vi "Periodic Tasks.vi"(8 "error in":errorcluster) -> ()   [LabVIEW 2015]
doc: "This VI runs in parallel to other tasks. It can contain as many user-defined periodic loops as you need. These can carry out PID or other sorts of timed response."
uses:
  <vilib>/Rock Robotics/SystemInterfaces/Utilities/FPGA_UtilitiesLED Source.ctl
  <vilib>/Rock Robotics/SystemInterfaces/Utilities/FPGA_UtilitiesLED State.ctl
  Robot Global Data.vi
  <vilib>/Rock Robotics/WPI/Solenoid/WPI_SolenoidValue.ctl
  <vilib>/Rock Robotics/WPI/Solenoid/WPI_SolenoidSetEnum.vi
panel:
  out "Enabled":bool
  out "Compressor Running":bool
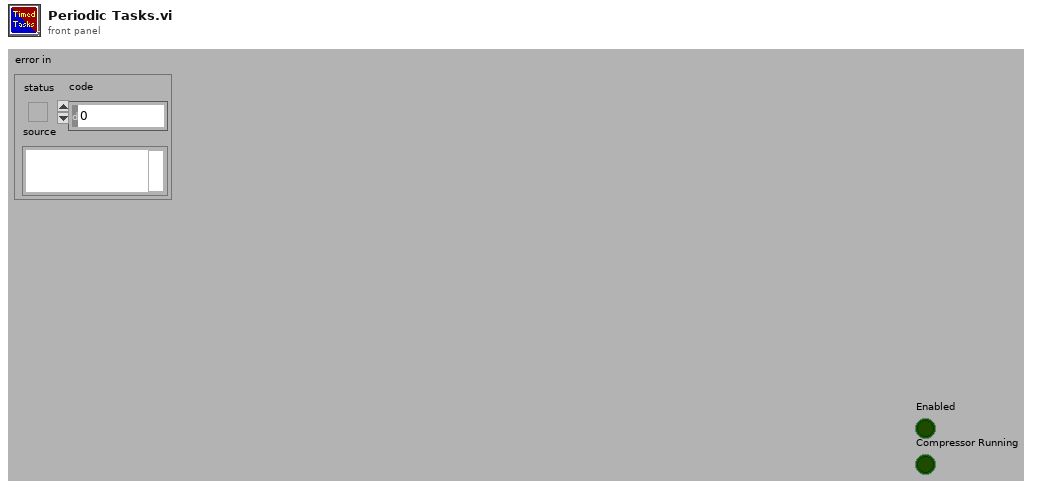
[diagram p1: front panel]
types:
  T1 = typedef "FPGA_UtilitiesLED State.ctl" = enum16{"Off", "On", "Toggle"}
  T2 = typedef "FPGA_UtilitiesLED Source.ctl" = enum16{"User LED", "FPGA LED"}
  T3 = typedef "WPI_MotorControlDeviceRef.ctl" = cluster{"DeviceStatus":errorcluster, "Type":enum16{"PWM", "CAN"}, "PWM":cluster{"Digital Module":T4, "PWM Channel":T5, "DeadBand":T6}, "CAN":cluster{"Device Number":u8, "Control Mode":T7, "Semaphore":T8, "Max Vout":dbl}, "Invert":bool, "TransformRef":T9, "InvTransformRef":T9}
  T4 = typedef "FPGA_TypedefDigitalModule.ctl" = enum16{"Digital Module 1", "Digital Module 2"}
  T5 = typedef "FPGA_DIOPWMChannel.ctl" = enum8{"PWM 1", "PWM 2", "PWM 3", "PWM 4", "PWM 5", "PWM 6", "PWM 7", "PWM 8", "PWM 9", "PWM 10", "Invalid"}
  T6 = typedef "WPI_PWMDeadband.ctl" = cluster{"Name":string, "maxPositivePwm":i32, "minPositivePwm":i32, "centerPwm":i32, "maxNegativePwm":i32, "minNegativePwm":i32, "angularRange":u16}
  T7 = typedef "WPI_CANJaguar_ControlMode.ctl" = enum8{"Percent VBus", "Current", "Speed", "Position", "Voltage"}
  T8 = typedef "Semaphore RefNum" = refnum<k1>
  T9 = typedef "WPI_PWMTransform_ConPane.ctl" = refnum<vi>
  T10 = typedef "WPI_SolenoidValue.ctl" = enum16{"Off", "On", "Forward", "Reverse"}
  T11 = typedef "WPI_SolenoidDevRef.ctl" = cluster{"DevStatus":errorcluster, "Solenoid Module":T12, "Forward Solenoid Channel":T13, "Reverse Solenoid Channel":T13}
  T12 = typedef "FPGA_TypedefSolenoidModule.ctl" = enum16{"Solenoid Module 1", "Solenoid Module 2"}
  T13 = typedef "WPI_SolenoidChannel.ctl" = enum8{"Solenoid 1", "Solenoid 2", "Solenoid 3", "Solenoid 4", "Solenoid 5", "Solenoid 6", "Solenoid 7", "Solenoid 8", "Invalid"}
  T14 = typedef "WPI_DriverStationRobotMode2.ctl" = enum16{"Autonomous Disabled", "Autonomous Enabled", "Teleop Disabled", "Teleop Enabled", "Disconnected", "Finish", "Test Disabled", "Test Enabled"}
  T15 = typedef "WPI_CompressorDevRef.ctl" = cluster{"DevStatus":errorcluster, "DigitalInputDevRef":T16, "RelayDevRef":T18}
  T16 = typedef "WPI_DigitalInputDevRef.ctl" = cluster{"DevStatus":errorcluster, "DIO Channel":T17, "Digital Module":T4}
  T17 = typedef "FPGA_DIOChannel.ctl" = enum8{"DIO 1", "DIO 2", "DIO 3", "DIO 4", "DIO 5", "DIO 6", "DIO 7", "DIO 8", "DIO 9", "DIO 10", "DIO 11", "DIO 12", "DIO 13", "DIO 14", "Invalid"}
  T18 = typedef "WPI_RelayDevRef.ctl" = cluster{"DevStatus":errorcluster, "Relay Channel":T19, "Digital Module":T4, "Relay Direction":T20}
  T19 = typedef "FPGA_DIORelayChannel.ctl" = enum8{"Relay 1", "Relay 2", "Relay 3", "Relay 4", "Relay 5", "Relay 6", "Relay 7", "Relay 8", "Invalid"}
  T20 = typedef "WPI_RelayDirection.ctl" = enum16{"Both directions", "Forward only", "Reverse only"}
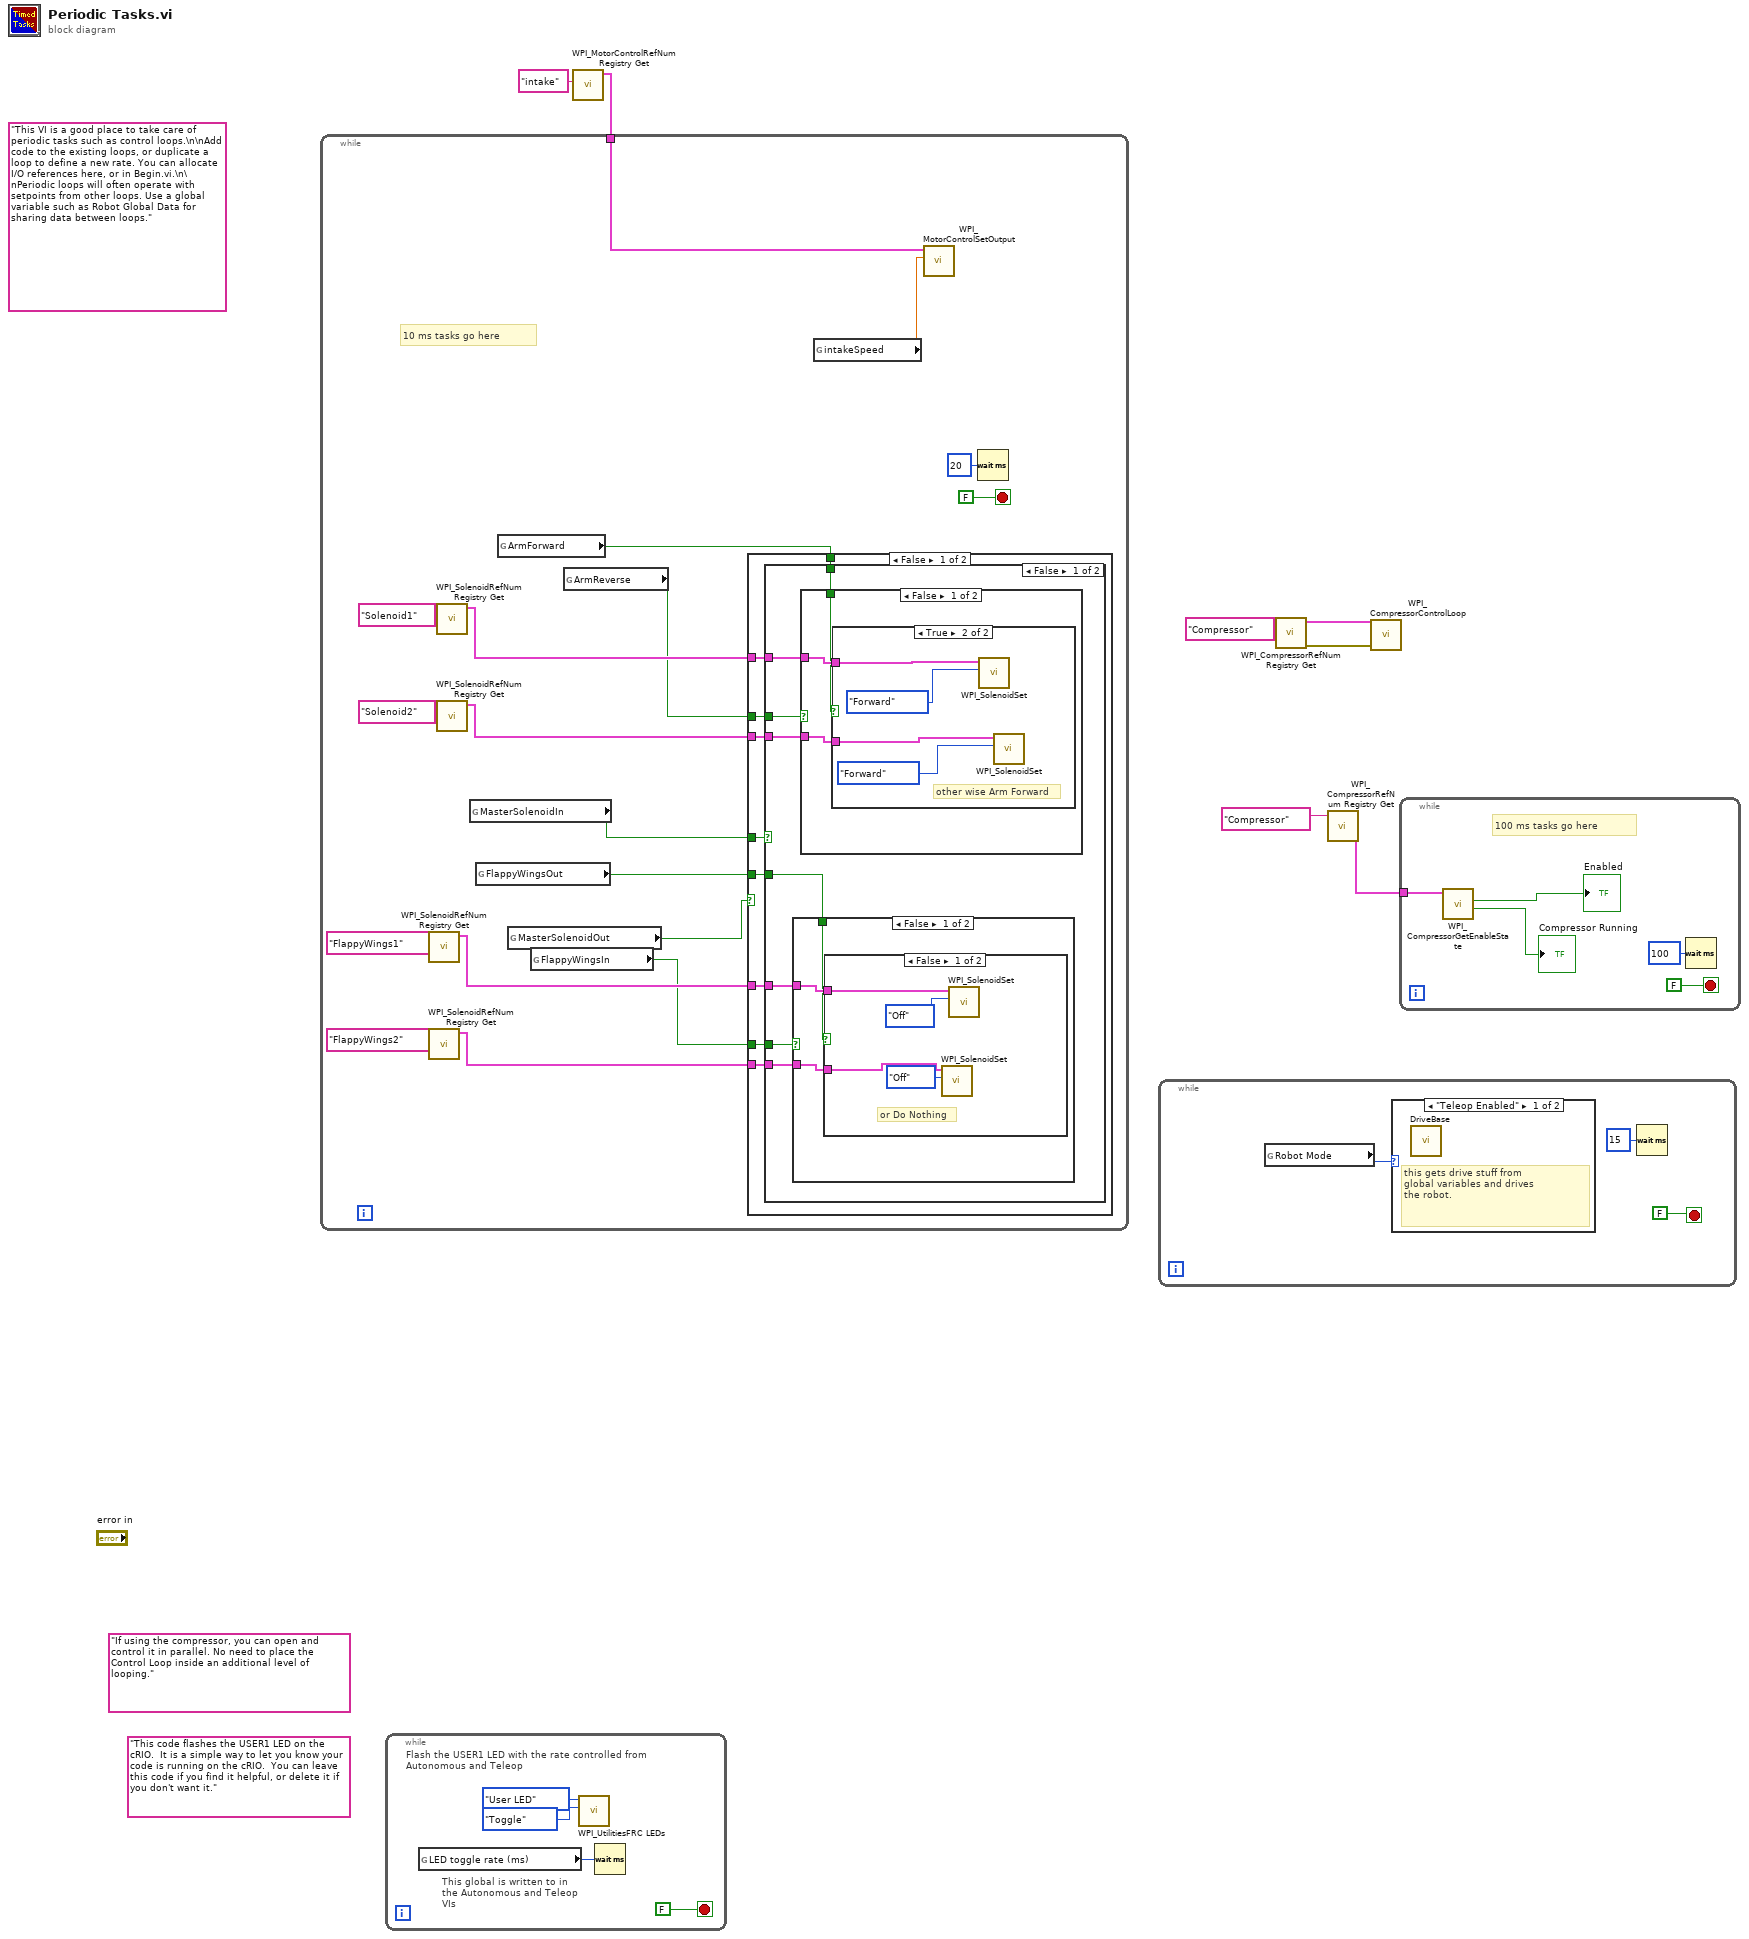
[diagram p0: block diagram]
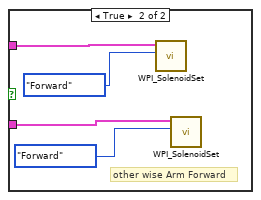
[diagram p2: hidden frame]
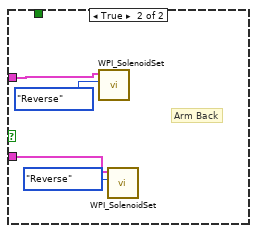
[diagram p3: hidden frame]
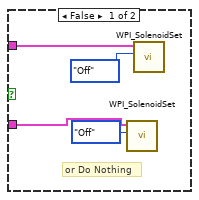
[diagram p4: hidden frame]
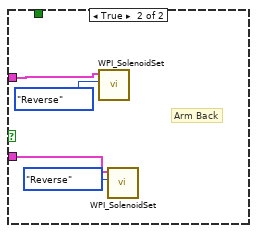
[diagram p5: hidden frame]
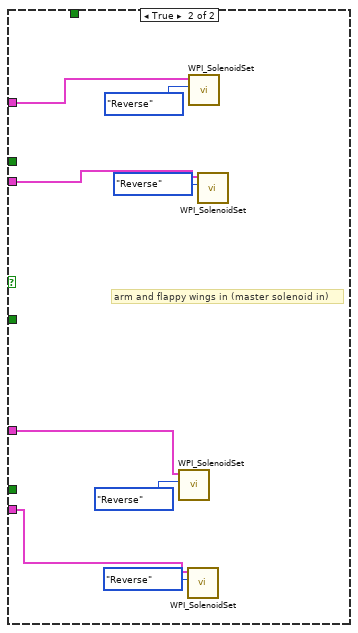
[diagram p6: hidden frame]
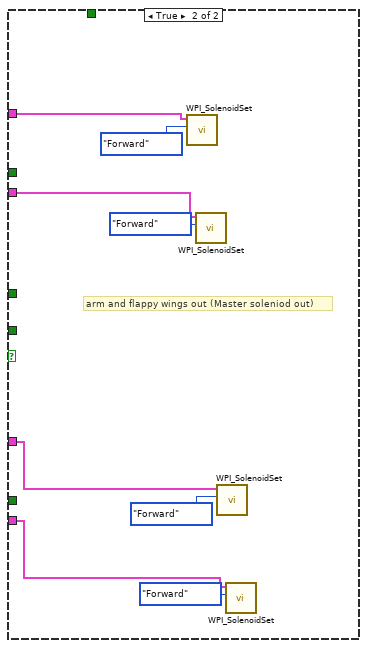
[diagram p7: hidden frame]
diagram:
  (unwired) "If using the compressor, you can open and control it in parallel. No need to place the Control Loop inside an additional level of looping."
  (unwired) "This code flashes the USER1 LED on the cRIO.  It is a simple way to let you know your code is running on the cRIO.  You can leave this code if you find it helpful, or delete it if you don't want it."
  (unwired) "This VI is a good place to take care of periodic tasks such as control loops.\n\nAdd code to the existing loops, or duplicate a loop to define a new rate. You can allocate I/O references here, or in Begin.vi.\n\nPeriodic loops will often operate with setpoints from other loops. Use a global variable such as Robot Global Data for sharing data between loops."
  n1 = while {
    stop <- FALSE stop-if-true
    # "This global is written to in the Autonomous and Teleop VIs"
    # "Flash the USER1 LED with the rate controlled from Autonomous and Teleop"
    n2 = global read "Robot Global Data.vi" "LED toggle rate (ms)"() -> (w8:u32)
    n3 = call <vilib>:"WPI_UtilitiesFRC LEDs.vi"("State"=FPGA_UtilitiesLED_State."Toggle", "LED Type"=FPGA_UtilitiesLED_Source."User LED") -> ()  [unwired: 1 in, 9 out]
    n4 = Wait (ms)(milliseconds to wait=w8) -> ()  [unwired: 1 out]
  }
  n5 = call <vilib>:"WPI_MotorControlRefNum Registry Get.vi"("refnum name"="intake") -> ("MotorControlDevRef"=w7:T3)  [unwired: 9 in, 1 out]
  n6 = while {
    tunnel: w7 -> [w27]
    stop <- FALSE stop-if-true
    # "10 ms tasks go here"
    n7 = call <vilib>:"WPI_SolenoidRefNum Registry Get.vi"("refnum name"="FlappyWings1") -> ("SolenoidDevRef"=w17:T11)  [unwired: 9 in, 1 out]
    n8 = call <vilib>:"WPI_SolenoidRefNum Registry Get.vi"("refnum name"="FlappyWings2") -> ("SolenoidDevRef"=w16:T11)  [unwired: 9 in, 1 out]
    n9 = call <vilib>:"WPI_SolenoidRefNum Registry Get.vi"("refnum name"="Solenoid1") -> ("SolenoidDevRef"=w23:T11)  [unwired: 9 in, 1 out]
    n10 = call <vilib>:"WPI_SolenoidRefNum Registry Get.vi"("refnum name"="Solenoid2") -> ("SolenoidDevRef"=w22:T11)  [unwired: 9 in, 1 out]
    n11 = global read "Robot Global Data.vi" "MasterSolenoidIn"() -> (w13:bool)
    n12 = global read "Robot Global Data.vi" "FlappyWingsOut"() -> (w15:bool)
    n13 = global read "Robot Global Data.vi" "ArmForward"() -> (w21:bool)
    n14 = global read "Robot Global Data.vi" "MasterSolenoidOut"() -> (w12:bool)
    n15 = global read "Robot Global Data.vi" "FlappyWingsIn"() -> (w14:bool)
    n16 = global read "Robot Global Data.vi" "ArmReverse"() -> (w20:bool)
    n17 = case shown="False" w12 {
      tunnel: w23 -> [w38 w90]
      tunnel: w22 -> [w37 w89]
      tunnel: w21 -> [w36 _]
      tunnel: w20 -> [w35 _]
      tunnel: w17 -> [w34 w85]
      tunnel: w16 -> [w33 w86]
      tunnel: w15 -> [w32 _]
      tunnel: w14 -> [w31 _]
      tunnel: w13 -> [w30 _]
      frame False {
        n18 = case shown="False" w30 {
          tunnel: w38 -> [w46 w81]
          tunnel: w37 -> [w45 w82]
          tunnel: w36 -> [w44 _]
          tunnel: w35 -> [w43 _]
          tunnel: w34 -> [w42 w78]
          tunnel: w33 -> [w41 w77]
          tunnel: w32 -> [w40 _]
          tunnel: w31 -> [w39 _]
          frame False {
            n19 = case shown="False" w39 {
              tunnel: w42 -> [w49 w61]
              tunnel: w41 -> [w48 w60]
              tunnel: w40 -> [w47 _]
              frame False {
                n20 = case shown="False" w47 {
                  tunnel: w49 -> [w52 w57]
                  tunnel: w48 -> [w50 w56]
                  frame False {
                    # "or Do Nothing"
                    n21 = call-poly <vilib>:"WPI_SolenoidSet.vi"("Value"=WPI_SolenoidValue."Off", "SolenoidDevRef"=w50) -> ()  [unwired: 8 in, 2 out]
                    n22 = call-poly <vilib>:"WPI_SolenoidSet.vi"("Value"=WPI_SolenoidValue."Off", "SolenoidDevRef"=w52) -> ()  [unwired: 8 in, 2 out]
                  }
                  frame True {
                    # "other wise Arm Forward"
                    n23 = call-poly <vilib>:"WPI_SolenoidSet.vi"("Value"=WPI_SolenoidValue."Forward", "SolenoidDevRef"=w57) -> ()  [unwired: 8 in, 2 out]
                    n24 = call-poly <vilib>:"WPI_SolenoidSet.vi"("Value"=WPI_SolenoidValue."Forward", "SolenoidDevRef"=w56) -> ()  [unwired: 8 in, 2 out]
                  }
                }
              }
              frame True {
                # "Arm Back"
                n25 = call-poly <vilib>:"WPI_SolenoidSet.vi"("Value"=WPI_SolenoidValue."Reverse", "SolenoidDevRef"=w61) -> ()  [unwired: 8 in, 2 out]
                n26 = call-poly <vilib>:"WPI_SolenoidSet.vi"("Value"=WPI_SolenoidValue."Reverse", "SolenoidDevRef"=w60) -> ()  [unwired: 8 in, 2 out]
              }
            }
            n27 = case shown="False" w43 {
              tunnel: w46 -> [w64 w76]
              tunnel: w45 -> [w63 w75]
              tunnel: w44 -> [w62 _]
              frame False {
                n28 = case shown="True" w62 {
                  tunnel: w64 -> [w67 w72]
                  tunnel: w63 -> [w65 w71]
                  frame False {
                    # "or Do Nothing"
                    n29 = call-poly <vilib>:"WPI_SolenoidSet.vi"("Value"=WPI_SolenoidValue."Off", "SolenoidDevRef"=w65) -> ()  [unwired: 8 in, 2 out]
                    n30 = call-poly <vilib>:"WPI_SolenoidSet.vi"("Value"=WPI_SolenoidValue."Off", "SolenoidDevRef"=w67) -> ()  [unwired: 8 in, 2 out]
                  }
                  frame True {
                    # "other wise Arm Forward"
                    n31 = call-poly <vilib>:"WPI_SolenoidSet.vi"("Value"=WPI_SolenoidValue."Forward", "SolenoidDevRef"=w72) -> ()  [unwired: 8 in, 2 out]
                    n32 = call-poly <vilib>:"WPI_SolenoidSet.vi"("Value"=WPI_SolenoidValue."Forward", "SolenoidDevRef"=w71) -> ()  [unwired: 8 in, 2 out]
                  }
                }
              }
              frame True {
                # "Arm Back"
                n33 = call-poly <vilib>:"WPI_SolenoidSet.vi"("Value"=WPI_SolenoidValue."Reverse", "SolenoidDevRef"=w76) -> ()  [unwired: 8 in, 2 out]
                n34 = call-poly <vilib>:"WPI_SolenoidSet.vi"("Value"=WPI_SolenoidValue."Reverse", "SolenoidDevRef"=w75) -> ()  [unwired: 8 in, 2 out]
              }
            }
          }
          frame True {
            # "arm and flappy wings in (master solenoid in)"
            n35 = call-poly <vilib>:"WPI_SolenoidSet.vi"("Value"=WPI_SolenoidValue."Reverse", "SolenoidDevRef"=w78) -> ()  [unwired: 8 in, 2 out]
            n36 = call-poly <vilib>:"WPI_SolenoidSet.vi"("Value"=WPI_SolenoidValue."Reverse", "SolenoidDevRef"=w77) -> ()  [unwired: 8 in, 2 out]
            n37 = call-poly <vilib>:"WPI_SolenoidSet.vi"("Value"=WPI_SolenoidValue."Reverse", "SolenoidDevRef"=w81) -> ()  [unwired: 8 in, 2 out]
            n38 = call-poly <vilib>:"WPI_SolenoidSet.vi"("Value"=WPI_SolenoidValue."Reverse", "SolenoidDevRef"=w82) -> ()  [unwired: 8 in, 2 out]
          }
        }
      }
      frame True {
        # "arm and flappy wings out (Master soleniod out)"
        n39 = call-poly <vilib>:"WPI_SolenoidSet.vi"("Value"=WPI_SolenoidValue."Forward", "SolenoidDevRef"=w90) -> ()  [unwired: 8 in, 2 out]
        n40 = call-poly <vilib>:"WPI_SolenoidSet.vi"("Value"=WPI_SolenoidValue."Forward", "SolenoidDevRef"=w89) -> ()  [unwired: 8 in, 2 out]
        n41 = call-poly <vilib>:"WPI_SolenoidSet.vi"("Value"=WPI_SolenoidValue."Forward", "SolenoidDevRef"=w85) -> ()  [unwired: 8 in, 2 out]
        n42 = call-poly <vilib>:"WPI_SolenoidSet.vi"("Value"=WPI_SolenoidValue."Forward", "SolenoidDevRef"=w86) -> ()  [unwired: 8 in, 2 out]
      }
    }
    n43 = global read "Robot Global Data.vi" "intakeSpeed"() -> (w26:dbl)
    n44 = call <vilib>:"WPI_MotorControlSetOutput.vi"("Output"=w26, "MotorControlDevRef"=w27) -> ()  [unwired: 7 in, 3 out]
    n45 = Wait (ms)(milliseconds to wait=u32 20) -> ()  [unwired: 1 out]
  }
  n46 = while {
    stop <- FALSE stop-if-true
    n47 = global read "Robot Global Data.vi" "Robot Mode"() -> (w93:T14)
    n48 = case shown="\"Teleop Enabled\"" w93 {
      frame "Teleop Enabled" {
        # "this gets drive stuff from\nglobal variables and drives \nthe robot."
        n49 = call "DriveBase.vi"() -> ()  [unwired: 12 in]
      }
      frame "Autonomous Disabled", Default {
      }
    }
    n50 = Wait (ms)(milliseconds to wait=u32 15) -> ()  [unwired: 1 out]
  }
  n51 = call <vilib>:"WPI_CompressorRefNum Registry Get.vi"("refnum name"="Compressor") -> ("error out"=w3:errorcluster, "CompressorDevRef"=w1:T15)  [unwired: 9 in]
  n52 = call <vilib>:"WPI_CompressorRefNum Registry Get.vi"("refnum name"="Compressor") -> ("CompressorDevRef"=w5:T15)  [unwired: 9 in, 1 out]
  n53 = call <vilib>:"WPI_CompressorControlLoop.vi"("error in (no error)"=w3, "CompressorDevRef"=w1) -> ()  [unwired: 10 in]
  n54 = while {
    tunnel: w5 -> [w98]
    stop <- FALSE stop-if-true
    # "100 ms tasks go here"
    n55 = call <vilib>:"WPI_CompressorGetEnableState.vi"("CompressorDevRef"=w98) -> ("Compressor Running"=→"Compressor Running":bool, "Enabled"=→"Enabled":bool)  [unwired: 7 in, 2 out]
    n56 = Wait (ms)(milliseconds to wait=u32 100) -> ()  [unwired: 1 out]
  }
